vi "fetch_and_translate_trigger.vi"(8 "error in (no error)":errorcluster, 11 "Stimulator090724Scaffold in":refnum<class "Stimulator090724Scaffold.lvclass">) -> (0 "error out":errorcluster, 1 "sender TLC type":T1=enum."ImagingMode", 2 "statechart trigger":T2, 3 "Stimulator090724Scaffold out":refnum<class "Stimulator090724Scaffold.lvclass">)   [LabVIEW 2010, in "Stimulator090724Scaffold.lvclass"]
uses:
  Stimulator090724Scaffold.lvclass
  internal_trigger_enum.ctl
  common/enumerations/top-level_component_type_enum.ctl
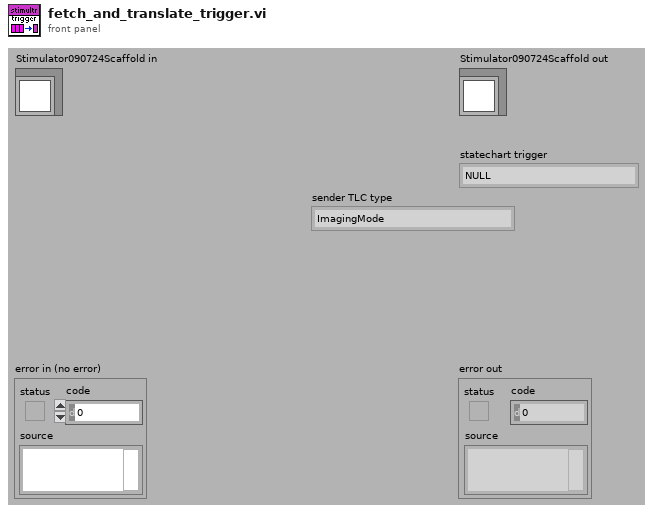
[diagram p1: front panel]
types:
  T1 = typedef "top-level_component_type_enum.ctl" = enum16{"undefined", "ImagingMode", "ScanHead", "DAQ", "ImageAssembler", "Display", "DataCollection", "Analyser", "Stimulator", "ExperimentController", "Instrument", "Stage"}
  T2 = typedef "Stimulator090724Scaffold.lvclass/internal_trigger_enum.ctl" = enum16{"NULL", "initialise", "terminate", "start sweep", "stop sweep", "start continuous stimulation", "stop continuous stimulation"}
  T3 = typedef "GenericToplevelComponent.lvclass/common_trigger_enum.ctl" = enum16{"NULL", "initialise", "terminate", "fetch command", "fetch data", "attach observer", "register as observer", "detach observer", "acknowledge", "start", "stop", "sweep started", "sweep finished", "experiment started", "experiment stopped"}
  T4 = typedef "trigger_type_enum.ctl" = enum8{"external", "internal", "common"}
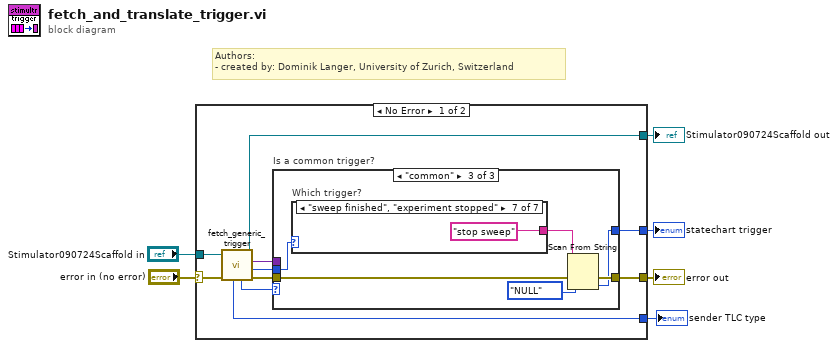
[diagram p0: block diagram]
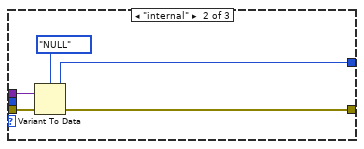
[diagram p3: hidden frame]
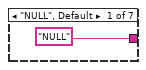
[diagram p4: hidden frame]
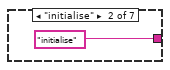
[diagram p5: hidden frame]
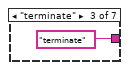
[diagram p6: hidden frame]
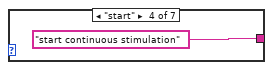
[diagram p7: hidden frame]
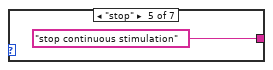
[diagram p8: hidden frame]
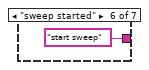
[diagram p9: hidden frame]
diagram:
  # "Authors: \n- created by: Dominik Langer, University of Zurich, Switzerland"
  n1 = case shown="No Error" "error in (no error)" {
    selector: "error in (no error)" -> [w14 w37]
    tunnel: [w16 w37] -> w5
    tunnel: [w10 w36] -> w3
    tunnel: "Stimulator090724Scaffold in" -> [w11 w36]
    tunnel: [w15 _] -> w1
    tunnel: [w7 _] -> w2
    frame No Error {
      n2 = call-dynamic "fetch_generic_trigger.vi"("error in (no error)"=w14, "GenericToplevelComponent in"=w11) -> ("error out"=w13:errorcluster, "common trigger"=w8:T3, "trigger"=w9:variant, "GenericToplevelComponent out"=w10:refnum<class "Stimulator090724Scaffold.lvclass">, "trigger type"=w12:T4, "sender TLC type"=w7:T1)  [unwired: 3 in, 1 out]
      n3 = case "Is a common trigger?" shown="\"common\"" w12 {
        tunnel: [w17 w21 w25] -> w16
        tunnel: [_ w19 w24] -> w15
        tunnel: w13 -> [w17 w22 w26]
        tunnel: w9 -> [_ w20 _]
        tunnel: w8 -> [_ _ w28]
        frame "external", Default {
          # "GenericStimulator does not provide external triggers."
        }
        frame "internal" {
          n4 = Variant To Data(error in=w22, Variant=w20, type=internal_trigger_enum."NULL" ("statechart trigger")) -> (error out=w21:errorcluster, data=w19:T2)
        }
        frame "common" {
          n5 = case "Which trigger?" shown="\"sweep finished\", \"experiment stopped\"" w28 {
            tunnel: ["NULL" "initialise" "terminate" "start continuous stimulation" "stop continuous stimulation" "start sweep" "stop sweep"] -> w23
            frame "NULL", Default {
            }
            frame "initialise" {
            }
            frame "terminate" {
            }
            frame "start" {
            }
            frame "stop" {
            }
            frame "sweep started" {
            }
            frame "sweep finished", "experiment stopped" {
            }
          }
          n6 = Scan From String(input string=w23, error in=w26, default 1=internal_trigger_enum."NULL" ("statechart trigger")) -> (error out=w25:errorcluster, output 1=w24:T2)  [unwired: 2 in, 2 out]
        }
      }
    }
    frame Error {
    }
  }
  "error out" <- w5
  "Stimulator090724Scaffold out" <- w3
  "statechart trigger" <- w1
  "sender TLC type" <- w2
